vi "Engine-Event-MouseWheel.vi"(4 "Mouse Position":T2, 6 "Wheel":T2, 7 "Mouse Wheel Direction":T1, 8 "error in (no error)":errorcluster, 9 "Which":T3, 10 "Timestamp":u64, 11 "GLF Window in":refnum<class "Window.lvclass">) -> (0 "error out":errorcluster, 3 "GLF Window out":refnum<class "Window.lvclass">)   [LabVIEW 2020, in "GLF.lvlib" / "Window.lvclass"]
uses:
  Window.lvclass
  Window.lvclass/Window.ctl
  WindowEventInterface/WindowEventInterface.lvclass
  <vilib>/Saukko/LV SDL3/Sources/SDL3/Mouse/MouseID--integer.ctl
  <vilib>/Saukko/LV SDL3/Sources/SDL3/Mouse/Mouse.lvlib
  <vilib>/Saukko/LV SDL3/Sources/SDL3/Rect/FPoint--cluster.ctl
  <vilib>/Saukko/LV SDL3/Sources/SDL3/Rect/Rect.lvlib
  <vilib>/Saukko/LV SDL3/Sources/SDL3/Mouse/MouseWheelDirection--enum.ctl
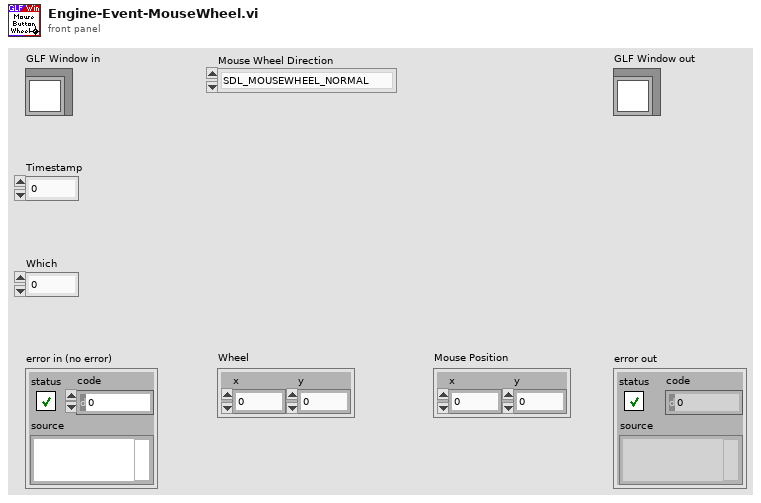
[diagram p1: front panel]
types:
  T1 = typedef "SDL3.lvlib/Mouse.lvlib/MouseWheelDirection--enum.ctl" = enum32{"SDL_MOUSEWHEEL_NORMAL", "SDL_MOUSEWHEEL_FLIPPED"}
  T2 = typedef "SDL3.lvlib/Rect.lvlib/FPoint--cluster.ctl" = cluster{"x":sgl, "y":sgl}
  T3 = typedef "SDL3.lvlib/Mouse.lvlib/MouseID--integer.ctl" = u32
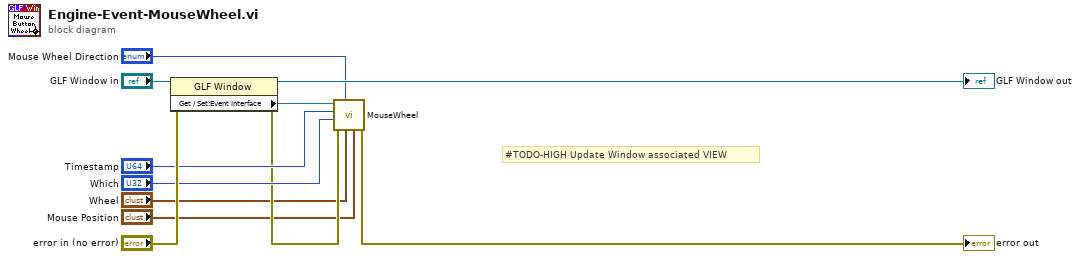
[diagram p0: block diagram]
diagram:
  # "#TODO-HIGH Update Window associated VIEW"
  n1 = property class="GLF Window"(reference="GLF Window in", error in="error in (no error)") -> (reference out=→"GLF Window out":refnum<class "Window.lvclass">, error out=w5:errorcluster, "Get / Set:Event Interface"=w9:refnum<class "WindowEventInterface.lvclass">)
  n2 = call-dynamic "MouseWheel.vi"("Mouse Position"="Mouse Position", "Wheel"="Wheel", "Mouse Wheel Direction"="Mouse Wheel Direction", "error in (no error)"=w5, "Which"="Which", "Timestamp"="Timestamp", "WindowEventInterface in"=w9) -> ("error out"=→"error out":errorcluster)  [unwired: 4 in]
